vi "mxwScript_Cmnd2Str_linkToPane.vi"(8 "error in (no error)":errorcluster, 11 "data":variant) -> (0 "error out":errorcluster, 3 "outputString":string)   [LabVIEW 2020]
uses:
  codeGenAPISupport.llb/cgAPI_mxwScript_LinkToPaneInfo.ctl
  codeGenAPISupport.llb/cgAPI_mxwScript_ConnPaneConnectionType.ctl
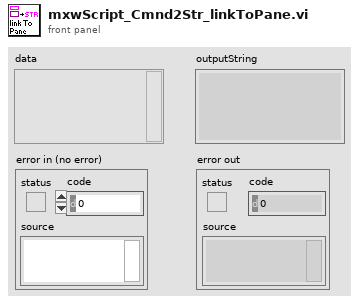
[diagram p1: front panel]
types:
  T1 = typedef "cgAPI_mxwScript_LinkToPaneInfo.ctl" = cluster{"controlName":string, "controlTemplateIndex":i32, "paneIndex":i32, "finalName":string, "connection type":T2}
  T2 = typedef "cgAPI_mxwScript_ConnPaneConnectionType.ctl" = enum16{"Invalid Wire Rule", "Required", "Recommended", "Optional", "Dynamic Dispatch"}
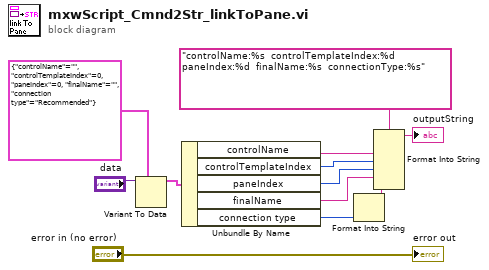
[diagram p0: block diagram]
diagram:
  n1 = Variant To Data(type=T1 {"controlName"="", "controlTemplateIndex"=0, "paneIndex"=0, "finalName"="", "connection type"=enum."Recommended"} ("linkToPaneInfo"), Variant="data") -> (data=w11:T1)  [unwired: 1 in, 1 out]
  n2 = Unbundle By Name(w11) -> ("controlName"=w7:string, "controlTemplateIndex"=w4:i32, "paneIndex"=w6:i32, "finalName"=w3:string, "connection type"=w2:T2)
  n3 = Format Into String(w2) -> (resulting string=w1:string)  [unwired: 3 in, 1 out]
  n4 = Format Into String(format string="controlName:%s  controlTemplateIndex:%d  paneIndex:%d  finalName:%s  connectionType:%s", w7, w4, w6, w3, w1) -> (resulting string=→"outputString":string)  [unwired: 2 in, 1 out]
  "error out" <- "error in (no error)"
